vi "OLD_Generate Tree from 2D Array of XML node paths.vi"(8 "error in (no error)":errorcluster, 10 "Array IN":string[][](array[string])=[["OME", "xsi:schemaLocation", "http://www.openmicroscopy.org/Schemas/OME/2015-01                         http://www.openmicroscopy.org/Schemas/OME/2015-01/ome.xsd", "", "", "", "", ""], ["OME", "Instrument", "ID", "Instrument:0", "", "", "", ""], ["OME", "Instrument", "Detector", "ID", "Detector:0:0", "", "", ""], ["OME", "Instrument", "Detector", "Model", "COOLSNAP_HQ / ICX285", "", "", ""], ["OME", "Instrument", "Detector", "Type", "CCD", "", "", ""], ["OME", "Instrument", "Objective", "ID", "Objective:10002", "", "", ""], ["OME", "Instrument", "Objective", "Immersion", "Water", "", "", ""], ["OME", "Instrument", "Objective", "LensNA", "1.4", "", "", ""], ["OME", "Instrument", "Objective", "Manufacturer", "Olympus", "", "", ""], ["OME", "Instrument", "Objective", "NominalMagnification", "100", "", "", ""], ["OME", "Image", "ID", "Default", "", "", "", ""], ["OME", "Image", "Name", "Default", "", "", "", ""], ["OME", "Image", "Pixels", "DimensionOrder", "XYCZT", "", "", ""], ["OME", "Image", "Pixels", "ID", "Pixels:0", "", "", ""], ["OME", "Image", "Pixels", "SizeC", "1", "", "", ""], ["OME", "Image", "Pixels", "SizeT", "10", "", "", ""], ["OME", "Image", "Pixels", "SizeX", "200", "", "", ""], ["OME", "Image", "Pixels", "SizeY", "200", "", "", ""], ["OME", "Image", "Pixels", "SizeZ", "5", "", "", ""], ["OME", "Image", "Pixels", "Type", "int8", "", "", ""], ["OME", "Image", "Pixels", "Channel", "ID", "Channel:1:2", "", ""], ["OME", "Image", "Pixels", "Channel", "IlluminationType", "Epifluorescence", "", ""], ["OME", "Image", "Pixels", "Channel", "NDFilter", "0.0", "", ""], ["OME", "Image", "Pixels", "Channel", "Name", "RD-TR-PE", "", ""], ["OME", "Image", "Pixels", "Channel", "SamplesPerPixel", "1", "", ""], ["OME", "Image", "SA:AnnotationRef", "ID", "Annotation:3", "", "", ""], ["OME", "SA:StructuredAnnotations", "SA:XMLAnnotation", "ID", "Annotation:3", "", "", ""], ["OME", "SA:StructuredAnnotations", "SA:XMLAnnotation", "Namespace", "openmicroscopy.org/omero/dimension/modulo", "", "", ""], ["OME", "SA:StructuredAnnotations", "SA:XMLAnnotation", "SA:Value", "Modulo", "namespace", "http://www.openmicroscopy.org/Schemas/Additions/2011-09", ""], ["OME", "SA:StructuredAnnotations", "SA:XMLAnnotation", "SA:Value", "Modulo", "ModuloAlongZ", "End", "580"], ["OME", "SA:StructuredAnnotations", "SA:XMLAnnotation", "SA:Value", "Modulo", "ModuloAlongZ", "Start", "480"], ["OME", "SA:StructuredAnnotations", "SA:XMLAnnotation", "SA:Value", "Modulo", "ModuloAlongZ", "Step", "25"], ["OME", "SA:StructuredAnnotations", "SA:XMLAnnotation", "SA:Value", "Modulo", "ModuloAlongZ", "Type", "phase"], ["OME", "SA:StructuredAnnotations", "SA:XMLAnnotation", "SA:Value", "Modulo", "ModuloAlongT", "Type", "lambda"]], 11 "Tree Refnum":refnum<vi>) -> (0 "error out":errorcluster)   [LabVIEW 2012]
doc: "SciScan 1.2 160622"
panel:
  out "Array":bool[](array[boolean])
  out "Array 3":u32[](array[numeric])
  out "Waveform Graph 2":u32[](graph)
  out "x/y 3":dbl
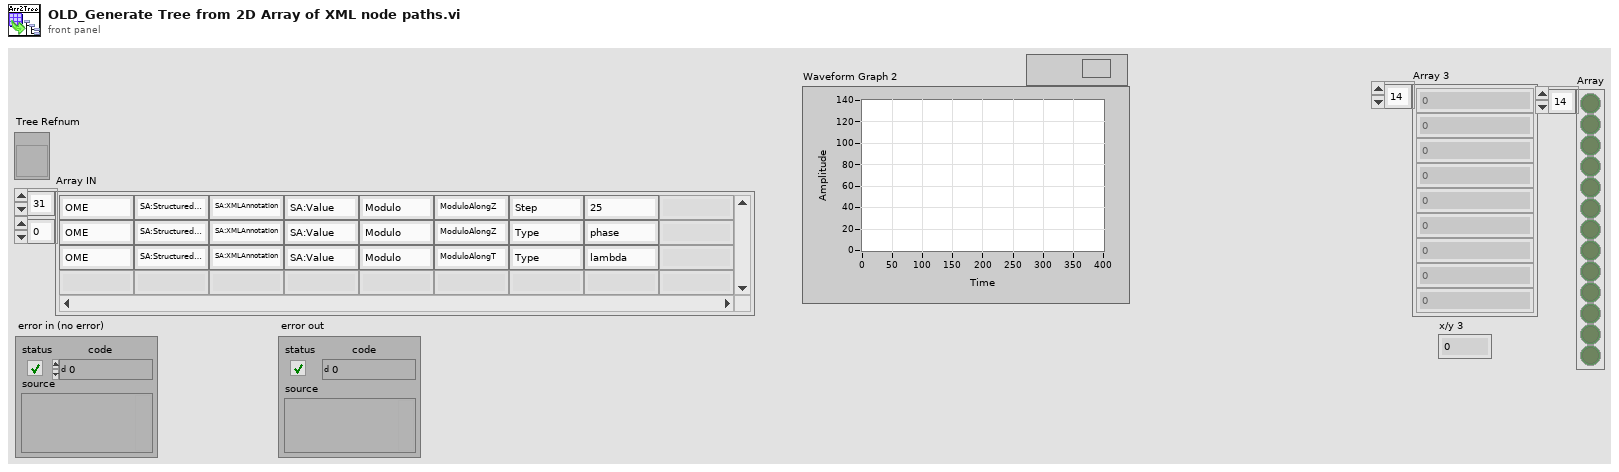
[diagram p1: front panel]
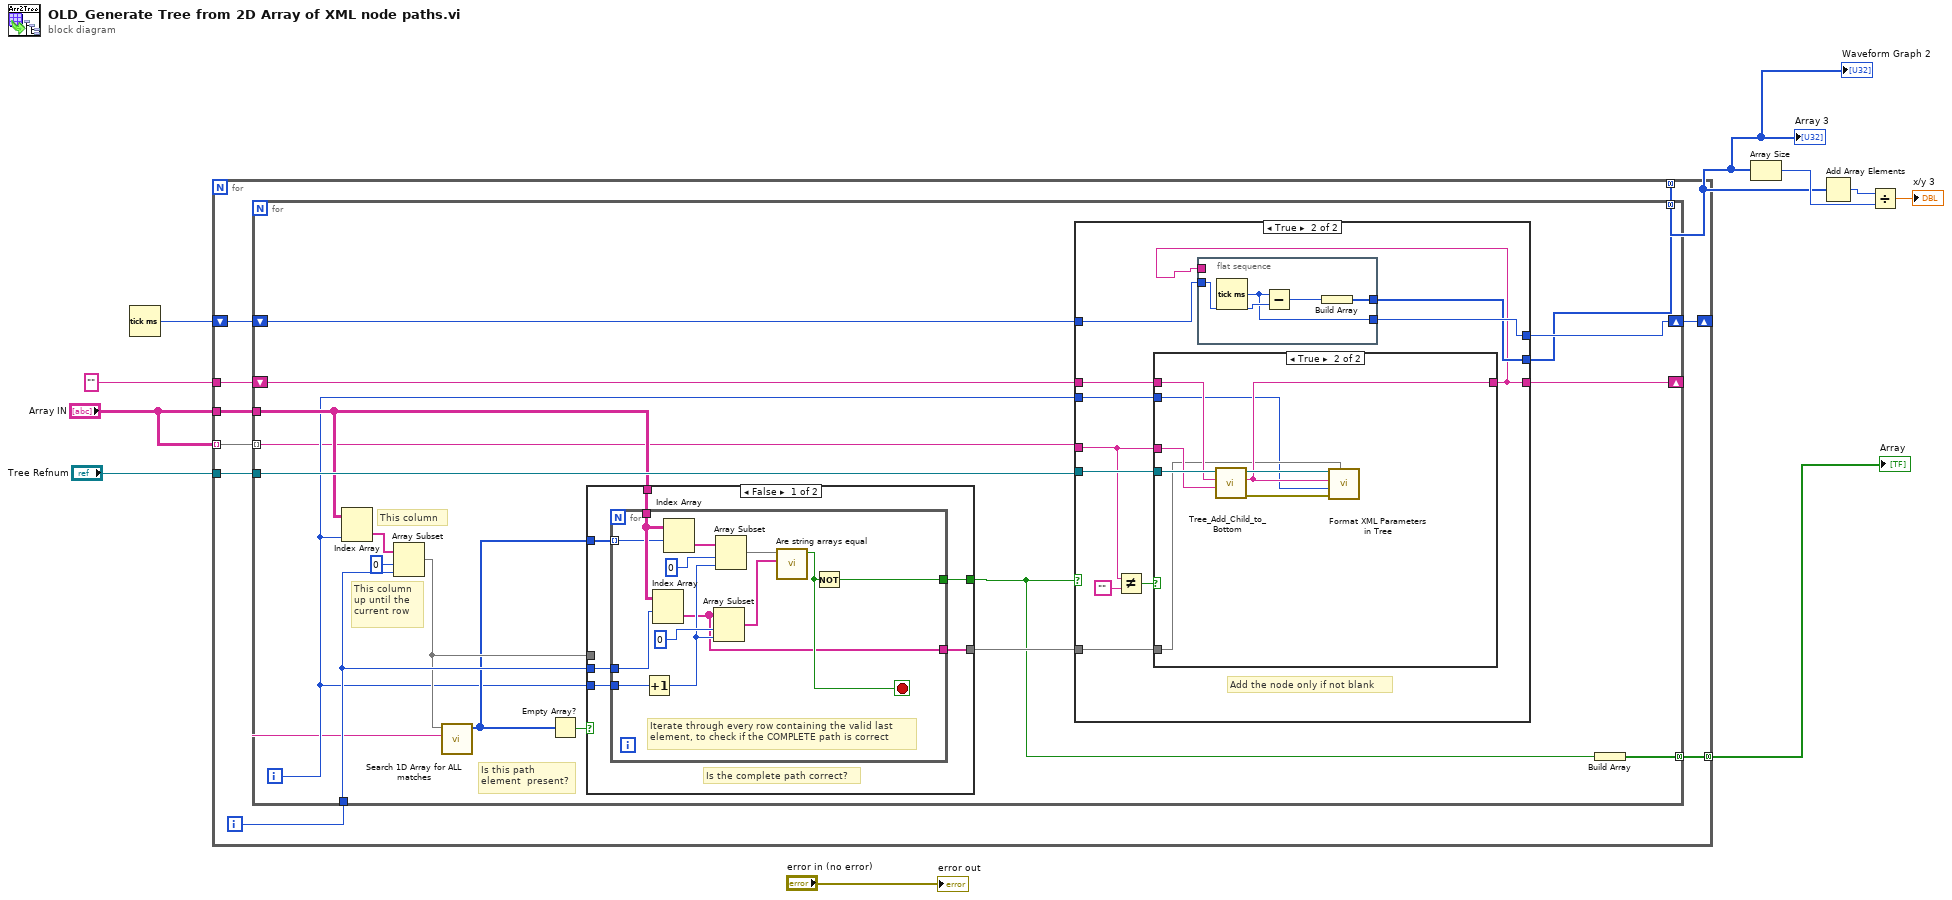
[diagram p0: block diagram]
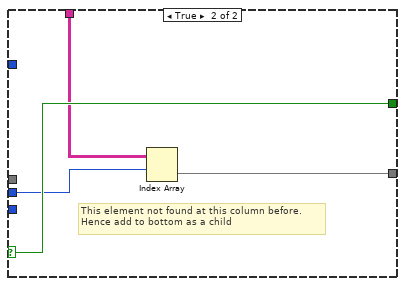
[diagram p2: hidden frame]
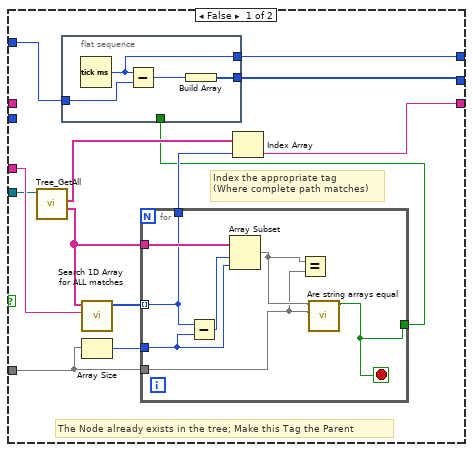
[diagram p3: hidden frame]
diagram:
  n1 = Tick Count (ms)() -> (millisecond timer value=w6:u32)
  n2 = for {
    tunnel: "Array IN" -> [w15] mode=indexing
    tunnel: "Tree Refnum" -> [w19]
    tunnel: "" -> [w18]
    tunnel: "Array IN" -> [w17]
    shift-right: [w12] -> _
    shift-left: w6 -> [w14]
    tunnel: [w13] -> w2 mode=concatenating
    tunnel: [w11] -> w1 mode=concatenating
    i -> [w16]
    n3 = for {
      tunnel: w15 -> [w27] mode=indexing
      tunnel: w19 -> [w36]
      shift-right: [w25] -> _
      shift-left: w18 -> [w37]
      tunnel: w17 -> [w33]
      tunnel: w16 -> [w32]
      shift-right: [w23] -> w12
      shift-left: w14 -> [w24]
      tunnel: [w22] -> w13 mode=concatenating
      tunnel: [w20] -> w11 mode=concatenating
      i -> [w28]
      # "This column up until the current row"
      # "This column"
      # "Is this path element  present?"
      n4 = Index Array(array=w33, index (col)=w28) -> (element=w35:string[])  [unwired: 1 in]
      n5 = Array Subset(array=w35, index=0, length=w32) -> (w31:string[])
      n6 = call "Search 1D Array for ALL matches.vi"("Se4arch string"=w27, "1D String Array"=w31) -> ("Found positions Array"=w29:i32[])  [unwired: 8 in, 1 out]
      n7 = Empty Array?(array=w29) -> (empty?=w30:bool)
      n8 = case shown="False" w30 {
        selector: w30 -> [_ w60]
        tunnel: [w39 w60] -> w21
        tunnel: w33 -> [w41 w59]
        tunnel: w32 -> [w42 w58]
        tunnel: w28 -> [w43 _]
        tunnel: w31 -> [_ _]
        tunnel: w29 -> [w40 _]
        tunnel: [w38 w57] -> w26
        frame False {
          # "Is the complete path correct?"
          n9 = for {
            tunnel: w43 -> [w56]
            tunnel: w42 -> [w55]
            tunnel: w41 -> [w51]
            tunnel: w40 -> [w50] mode=indexing
            tunnel: [w45] -> w39
            tunnel: [w44] -> w38
            stop <- w46 stop-if-true
            # "Iterate through every row containing the valid last\nelement, to check if the COMPLETE path is correct"
            n10 = Increment(x=w56) -> (x+1=w49:i32)
            n11 = Index Array(array=w51, index (row)=w55) -> (element=w44:string[])  [unwired: 1 in]
            n12 = Index Array(array=w51, index (row)=w50) -> (element=w52:string[])  [unwired: 1 in]
            n13 = Array Subset(array=w44, index=0, length=w49) -> (w47:string[])
            n14 = Array Subset(array=w52, index=0, length=w49) -> (w48:string[])
            n15 = call "Are string arrays equal.vi"("1D String Array 2"=w47, "1D String Array 1"=w48) -> ("EQUAL?"=w46:bool)  [unwired: 8 in, 1 out]
            n16 = Not(x=w46) -> (.not. x?=w45:bool)
          }
        }
        frame True {
          # "This element not found at this column before.\nHence add to bottom as a child"
          n17 = Index Array(array=w59, index (row)=w58) -> (element=w57:string[])  [unwired: 1 in]
        }
      }
      n18 = case shown="True" w21 {
        tunnel: w36 -> [w67 w95]
        tunnel: w27 -> [w72 w92]
        tunnel: [w73 w85] -> w25
        tunnel: w37 -> [_ w94]
        tunnel: w26 -> [w69 w90]
        tunnel: w28 -> [_ w89]
        tunnel: w24 -> [w63 w88]
        tunnel: [w62 w86] -> w22
        tunnel: [w61 w87] -> w23
        frame False {
          # "Index the appropriate tag\n(Where complete path matches)"
          # "The Node already exists in the tree; Make this Tag the Parent"
          n19 = call "Tree_GetAll.vi"("Tree Refnum IN"=w67) -> ("Text"=w65:string[], "Tags"=w66:string[])  [unwired: 7 in, 2 out]
          n20 = flat-sequence {
            tunnel: w63 -> [w76]
            tunnel: [w75] -> w62
            tunnel: [w74] -> w61
            tunnel: w64 -> [_]
            frame #0 {
              n21 = Tick Count (ms)() -> (millisecond timer value=w74:u32)
              n22 = Subtract(x=w74, y=w76) -> (x-y=w77:u32)
              n23 = Build Array(w77) -> (w75:u32[])
            }
          }
          n24 = call "Search 1D Array for ALL matches.vi"("Se4arch string"=w72, "1D String Array"=w65) -> ("Found positions Array"=w71:i32[])  [unwired: 8 in, 1 out]
          n25 = Array Size(array=w69) -> (size(s)=w70:i32)
          n26 = for {
            tunnel: w65 -> [w84]
            tunnel: w71 -> [w81] mode=indexing
            tunnel: w70 -> [w82]
            tunnel: w69 -> [w78]
            tunnel: [w81] -> w68
            tunnel: [w80] -> w64
            stop <- w80 stop-if-true
            n27 = Subtract(x=w81, y=w82) -> (x-y=w83:i32)
            n28 = Array Subset(array=w84, index=w83, length=w82) -> (w79:string[])
            n29 = Equal?(x=w79, y=w78) -> ()  [unwired: 1 out]
            n30 = call "Are string arrays equal.vi"("1D String Array 2"=w78, "1D String Array 1"=w79) -> ("EQUAL?"=w80:bool)  [unwired: 8 in, 1 out]
          }
          n31 = Index Array(array=w66, index=w68) -> (element=w73:string)
        }
        frame True {
          # "Add the node only if not blank"
          n32 = Not Equal?(x=w92, y="") -> (x != y?=w91:bool)
          n33 = case shown="True" w91 {
            tunnel: w95 -> [_ w108]
            tunnel: w94 -> [w100 w106]
            tunnel: w92 -> [_ w107]
            tunnel: [w100 w104] -> w85
            tunnel: w90 -> [_ w103]
            tunnel: w89 -> [_ w102]
            frame False {
            }
            frame True {
              n34 = call "Tree_Add_Child_to_Bottom.vi"("Child String (to add)"=w107, "Parent Tag"=w106, "Tree Refnum IN"=w108) -> ("error out"=w101:errorcluster, "Newly added Child Tag"=w104:string, "Tree Refnum OUT"=w105:refnum<vi>)  [unwired: 6 in]
              n35 = call "Format XML Parameters in Tree.vi"("Path  Array IN"=w103, "error in (no error)"=w101, "Current path index"=w102, "Newly Added Tag"=w104, "Tree Refnum"=w105) -> ()  [unwired: 7 in]
            }
          }
          n36 = flat-sequence {
            tunnel: [w98] -> w86
            tunnel: w88 -> [w97]
            tunnel: [w96] -> w87
            tunnel: w85 -> [_]
            frame #0 {
              n37 = Tick Count (ms)() -> (millisecond timer value=w96:u32)
              n38 = Subtract(x=w96, y=w97) -> (x-y=w99:u32)
              n39 = Build Array(w99) -> (w98:u32[])
            }
          }
        }
      }
      n40 = Build Array(w21) -> (w20:bool[])
    }
  }
  "Waveform Graph 2" <- w2
  "Array 3" <- w2
  "Array" <- w1
  n41 = Array Size(array=w2) -> (size(s)=w4:i32)
  n42 = Add Array Elements(numeric array=w2) -> (sum=w5:u32)
  n43 = Divide(x=w5, y=w4) -> (x/y=→"x/y 3":dbl)
  "error out" <- "error in (no error)"
